vi "New String Group.vi"(8 "error in (no error)":errorcluster, 10 "Group Config":refnum<class "Group Config.lvclass">, 11 "ChannelService in":refnum<class "ChannelService.lvclass">) -> (0 "error out":errorcluster, 2 "StringGroup":refnum<class "StringGroup.lvclass">, 3 "ChannelService out":refnum<class "ChannelService.lvclass">)   [LabVIEW 2020, in "Vecto.lvlib" / "ChannelService.lvclass"]
uses:
  ChannelService.lvclass
  Group Config/Group Config.lvclass
  StringGroup/StringGroup.lvclass
  C:/dev/lv20CE/relink/lv-vecto/Vecto/GroupAbstract/GroupAbstract.lvclass
  ChannelService.lvclass/ChannelService.ctl
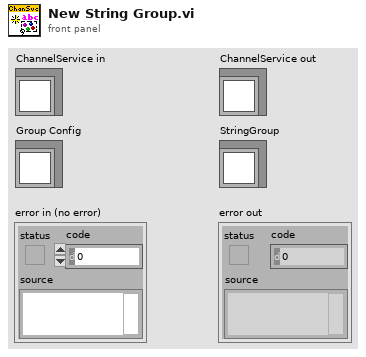
[diagram p1: front panel]
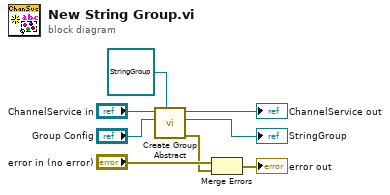
[diagram p0: block diagram]
diagram:
  n1 = call "Create Group Abstract.vi"("Group Type"=refnum<class "StringGroup.lvclass"> refnum ("StringGroup"), "Group Config"="Group Config", "ChannelService in"="ChannelService in") -> ("error out"=w1:errorcluster, "Group"=→"StringGroup":refnum<class "StringGroup.lvclass">, "ChannelService out"=→"ChannelService out":refnum<class "ChannelService.lvclass">)  [unwired: 6 in]
  n2 = Merge Errors("error in (no error)", w1) -> (→"error out":errorcluster)
